vi "Do.vi"(8 "error in (no error)":errorcluster, 10 "Actor in":refnum<class "Actor.lvclass">, 11 "Set OD Entry Values Msg":refnum<class "Set OD Entry Values Msg.lvclass">) -> (0 "error out":errorcluster, 2 "Actor out":refnum<class "Actor.lvclass">)   [LabVIEW 2024, in "Object Dictionary UI.lvlib" / "Set OD Entry Values Msg.lvclass"]
doc: "This VI delivers the message to the actor by calling the appropriate method(s) on the actor."
uses:
  Set OD Entry Values Msg.lvclass
  <vilib>/ActorFramework/Actor/Actor.lvclass
  Set OD Entry Values Msg.lvclass/Set OD Entry Values Msg.ctl
  Object Dictionary UI/Object Dictionary UI.lvclass
  C:/Program Files/National Instruments/LabVIEW 2025/vi.lib/ActorFramework/Actor/Actor.lvclass
  deab7600-629c-4f18-a0ba-4ada1eaa7511.vi
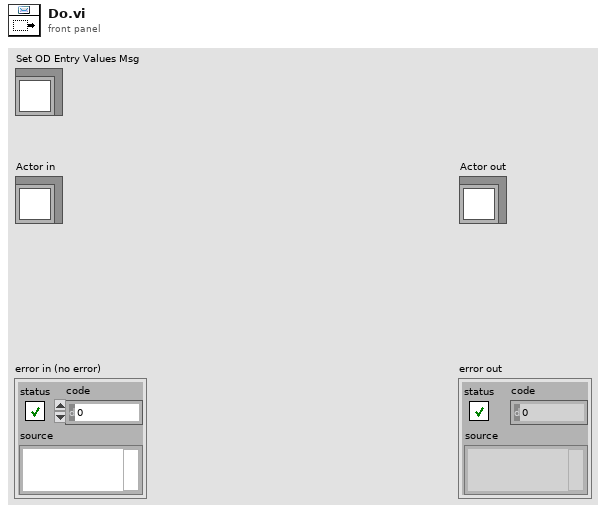
[diagram p1: front panel]
types:
  T1 = cluster{"Multiplexer":cluster{"Index":u16, "Sub-Index":u8}, "Value":u8[]}[]
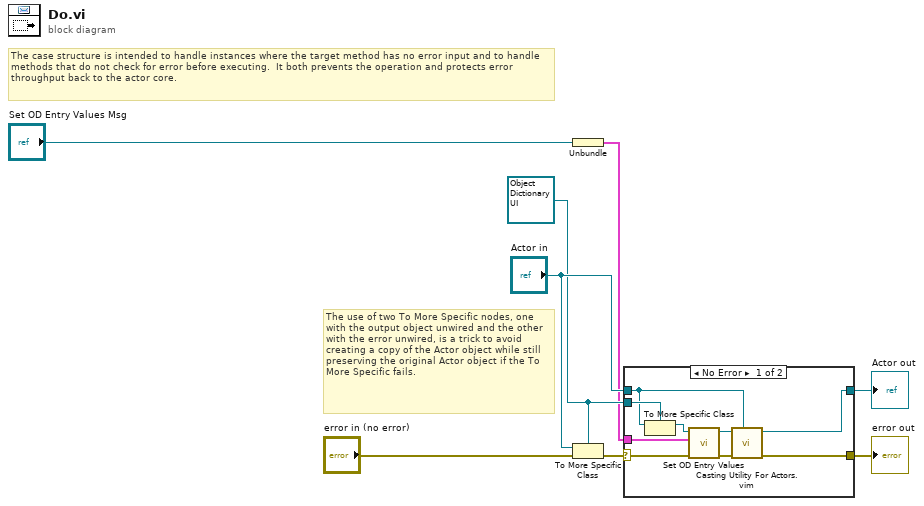
[diagram p0: block diagram]
diagram:
  w3 = refnum<class "Object Dictionary UI.lvclass"> refnum ("Actor in")
  # "The use of two To More Specific nodes, one with the output object unwired and the other with the error unwired, is a trick to avoid creating a copy of the Actor object while still preserving the original Actor object if the To More Specific fails."
  # "The case structure is intended to handle instances where the target method has no error input and to handle methods that do not check for error before executing.  It both prevents the operation and protects error throughput back to the actor core."
  n1 = Unbundle("Set OD Entry Values Msg") -> (w1:T1)
  n2 = To More Specific Class(target class=w3, reference="Actor in", error in="error in (no error)") -> (error out=w2:errorcluster)  [unwired: 1 out]
  n3 = case shown="No Error" w2 {
    selector: w2 -> [w17 w19]
    tunnel: [w11 w19] -> w8
    tunnel: [w12 w18] -> w7
    tunnel: "Actor in" -> [w14 w18]
    tunnel: w3 -> [w15 _]
    tunnel: w1 -> [w9 _]
    frame No Error {
      n4 = To More Specific Class(target class=w15, reference=w14) -> (specific class reference=w16:refnum<class "Object Dictionary UI.lvclass">)  [unwired: 1 in, 1 out]
      n5 = call-dynamic "Set OD Entry Values.vi"("error in"=w17, "Values"=w9, "Object Dictionary UI in"=w16) -> ("error out"=w10:errorcluster, "Object Dictionary UI out"=w13:refnum<class "Object Dictionary UI.lvclass">)  [unwired: 7 in]
      n6 = call "Casting Utility For Actors.vim"("type"=w14, "error in (no error)"=w10, "Actor in"=w13) -> ("error out"=w11:errorcluster, "Actor out"=w12:refnum<class "Actor.lvclass">)  [unwired: 7 in]
    }
    frame Error {
      # "If type check fails, pass the original object out again."
    }
  }
  "error out" <- w8
  "Actor out" <- w7
